vi "Connection Mode Generation Create New TP Connection.vi"(5 "Data to Send":T1 {"Identifier" format="%08x"}, 11 "error in (no error)":errorcluster) -> (4 "Connections Cluster":T2 {"Packets"."Identifier" format="%08x"}, 6 "Connection Management Packet":T1 {"Identifier" format="%08x"}, 15 "error out":errorcluster)   [LabVIEW 2015, in "J1939 Addon Engine.lvlib"]
uses:
  J1939 Addon Engine.lvlib
  Types/Connection Mode Generation Connection Cluster.ctl
  Shared/J1939 Utilities/Types/CAN Outgoing Message Cluster.ctl
  Shared/J1939 Utilities/SubVIs/Convert CAN Arb ID to J1939 ID.vi
  Shared/J1939 Utilities/SubVIs/TP.CM RTS.vi
  Shared/J1939 Utilities/SubVIs/TP.DT.vi
  Shared/J1939 Utilities/SubVIs/Convert J1939 ID to CAN Arb ID.vi
  Shared/J1939 Utilities/J1939 Utilities.lvlib
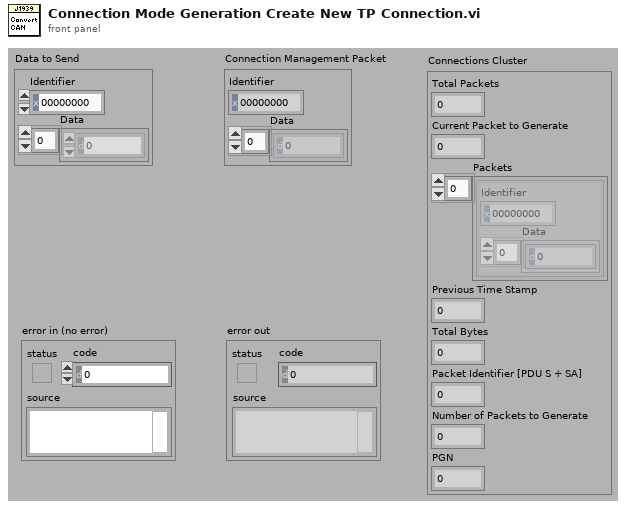
[diagram p1: front panel]
types:
  T1 = typedef "J1939 Addon Shared.lvlib/J1939 Utilities.lvlib/CAN Outgoing Message Cluster.ctl" = cluster{"Identifier":u32, "Data":u8[]}
  T2 = typedef "J1939 Addon Engine.lvlib/Connection Mode Generation Connection Cluster.ctl" = cluster{"Total Packets":u8, "Current Packet to Generate":u8, "Packets":T1[], "Previous Time Stamp":u32, "Total Bytes":u16, "Packet Identifier [PDU S + SA]":u16, "Number of Packets to Generate":u8, "PGN":u32}
  T3 = typedef "J1939 Addon Shared.lvlib/J1939 Utilities.lvlib/PGN Fields Cluster.ctl" = cluster{"Reserved Bit":u8, "Data page":u8, "PDU Format":u8, "PDU Specific":u8}
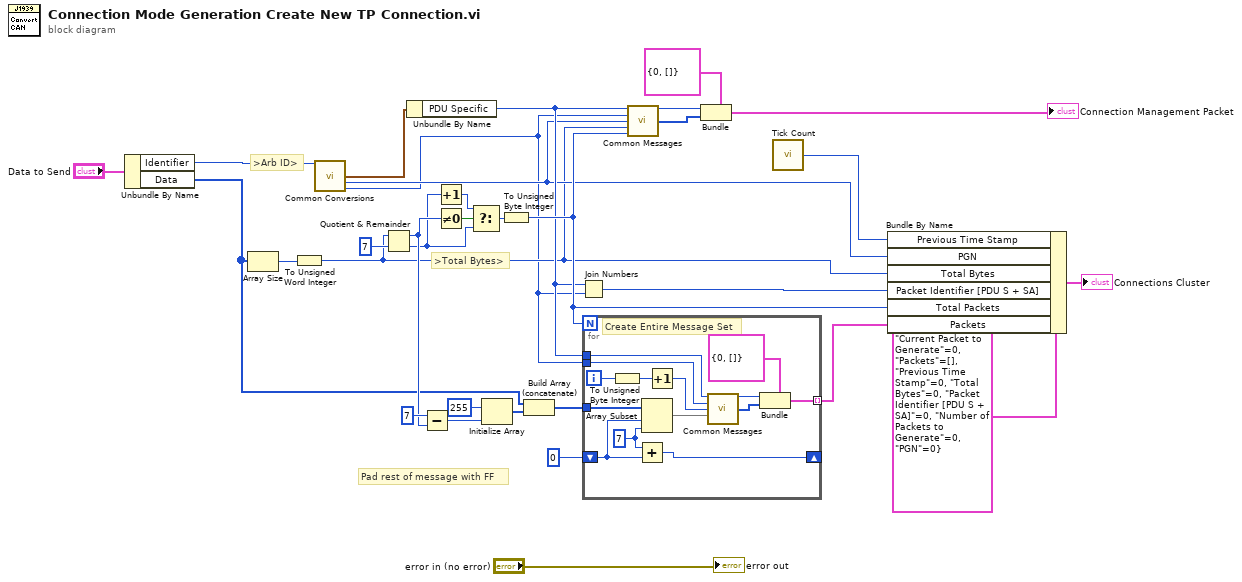
[diagram p0: block diagram]
diagram:
  # "Pad rest of message with FF"
  # ">Arb ID>"
  # ">Total Bytes>"
  n1 = Unbundle By Name("Data to Send") -> ("Identifier"=w9:u32, "Data"=w2:u8[])
  n2 = Array Size(array=w2) -> (size(s)=w14:i32)
  n3 = To Unsigned Word Integer(number=w14) -> (unsigned 16bit integer=w3:u16)
  n4 = call-poly "Common Conversions.vi"("Arb ID"=w9) -> ("PGN Fields"=w31:T3, "PGN"=w13:u32, "Source Address"=w1:u8)  [unwired: 12 out]
  n5 = Quotient & Remainder(x=w3, y=u16 7) -> (x-y*floor(x/y)=w25:u16, floor(x/y)=w21:u16)
  n6 = Unbundle By Name(w31) -> ("PDU Specific"=w15:u8)
  n7 = Subtract(x=u8 7, y=w25) -> (x-y=w27:u16)
  n8 = Increment(x=w21) -> (x+1=w20:u16)
  n9 = Not Equal To 0?(x=w25) -> (x != 0?=w19:bool)
  n10 = Select(t=w20, s=w19, f=w21) -> (s? t:f=w22:u16)
  n11 = Initialize Array(u8 255, w27) -> (w28:u8[])
  n12 = To Unsigned Byte Integer(number=w22) -> (unsigned 8bit integer=w16:u8)
  n13 = Build Array (concatenate)(w2, w28) -> (w29:u8[])
  n14 = Join Numbers(hi=w15, lo=w1) -> ((hi.lo)=w32:u16)
  n15 = for {
    N: w16 -> [_]
    tunnel: w29 -> [w46]
    shift-right: [w43] -> _
    shift-left: 0 ("index") -> [w44]
    tunnel: [w34] -> w8 mode=indexing
    tunnel: w1 -> [w39]
    tunnel: w15 -> [w40]
    i -> [w42]
    w45 = 7 ("length")
    # "Create Entire Message Set"
    n16 = To Unsigned Byte Integer(number=w42) -> (unsigned 8bit integer=w41:u8)
    n17 = Add(x=w45, y=w44) -> (x+y=w43:i32)
    n18 = Array Subset(array=w46, index=w44, length=w45) -> (w37:u8[])
    n19 = Increment(x=w41) -> (x+1=w38:u8)
    n20 = call-poly "Common Messages.vi"("Destination Address"=w40, "Source Address"=w39, "Sequence Number"=w38, "Data"=w37) -> ("Arb ID"=w36:u32, "Data"=w35:u8[])  [unwired: 10 out]
    n21 = Bundle(cluster=T1 {"Identifier"=0, "Data"=[]}, "Identifier"=w36, "Data"=w35) -> (w34:T1)
  }
  n22 = call-poly "Common Messages.vi"("Destination Address"=w15, "Source Address"=w1, "PGN"=w13, "Total Message Size(bytes)"=w3, "Total Number of Packets"=w16) -> ("Arb ID"=w12:u32, "Data"=w11:u8[])  [unwired: 9 out]
  n23 = Bundle(cluster=T1 {"Identifier"=0, "Data"=[]}, "Identifier"=w12, "Data"=w11) -> (→"Connection Management Packet":T1)
  n24 = call "Tick Count"() -> ("Tick Count(mSec)"=w5:u32)
  n25 = Bundle By Name(cluster=T2 {"Total Packets"=0, "Current Packet to Generate"=0, "Packets"=[], "Previous Time Stamp"=0, "Total Bytes"=0, "Packet Identifier [PDU S + SA]"=0, "Number of Packets to Generate"=0, "PGN"=0} ("Cluster"), "Previous Time Stamp"=w5, "PGN"=w13, "Total Bytes"=w3, "Packet Identifier [PDU S + SA]"=w32, "Total Packets"=w16, "Packets"=w8) -> (→"Connections Cluster":T2)
  "error out" <- "error in (no error)"
